vi "Universal_Stepping.vi"(7 "Initial Voltage (V)":dbl caption="Initial Value", 9 "Voltage Step (V)":dbl=0.01 caption="Step Value", 10 "Final Voltage (V)":dbl=0.1 caption="Final Value", 11 "VISA resource name":refnum<visa-resource-name>) -> (1 "Ready":bool, 2 "Actual Voltage (V)":dbl caption="Actual Value" step=0.1)   [LabVIEW 2015]
panel:
  in  "Command":string="smua.source.leveli="
  out "Visa Command":string
  out "Increase/Decrease":string
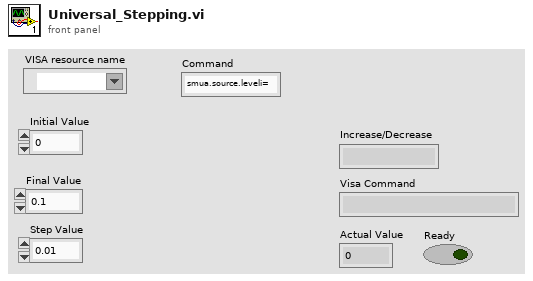
[diagram p1: front panel]
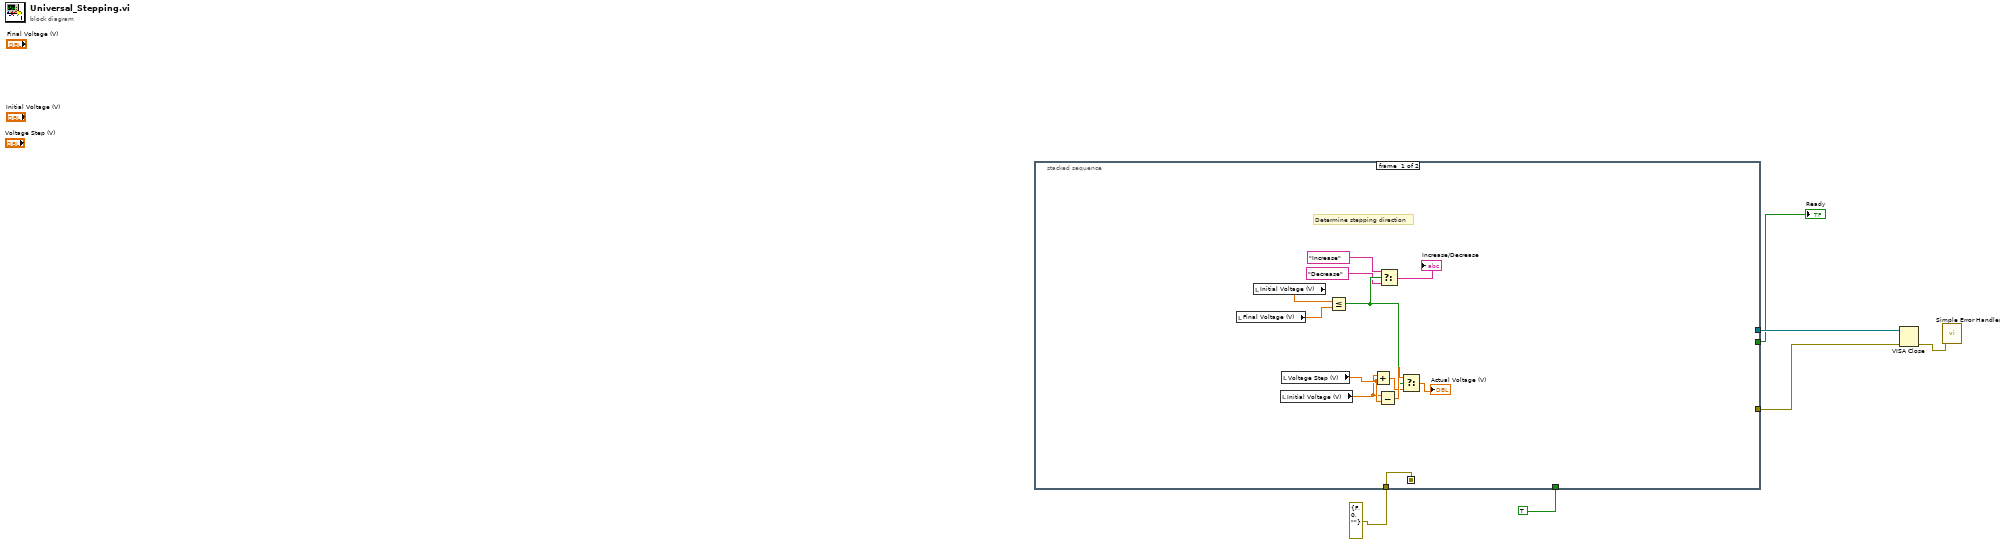
[diagram p0: block diagram]
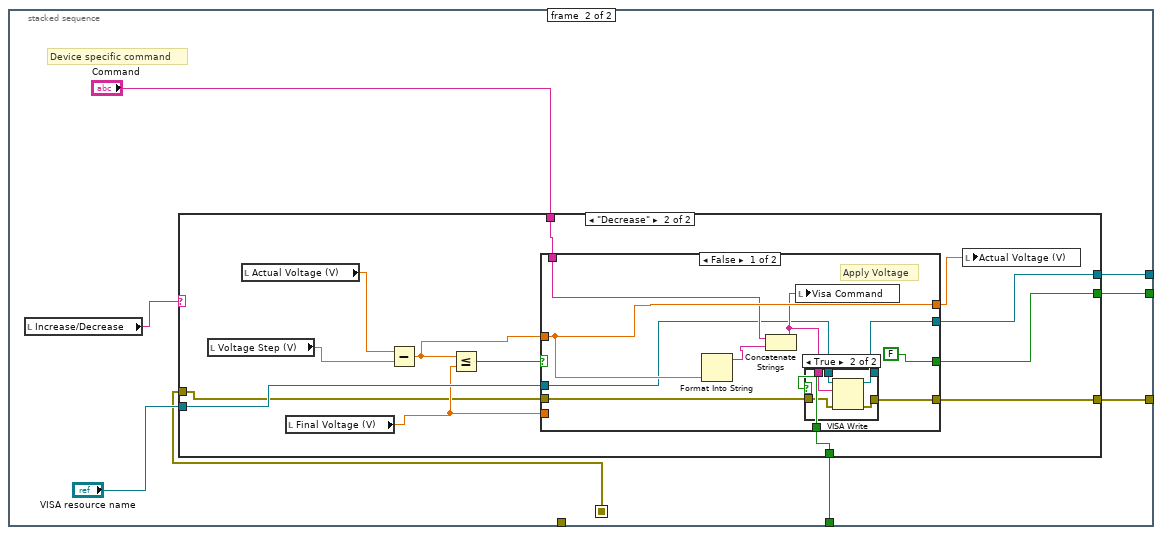
[diagram p2: hidden frame]
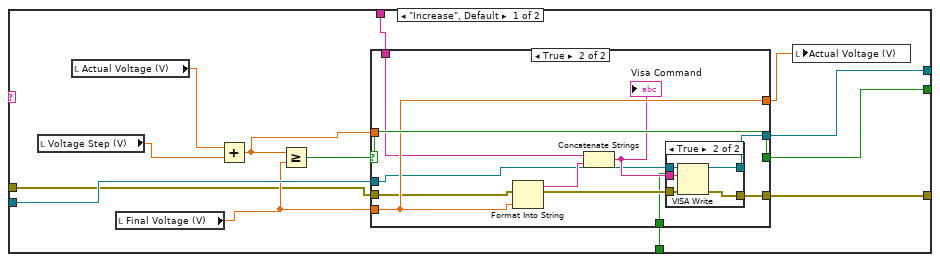
[diagram p3: hidden frame]
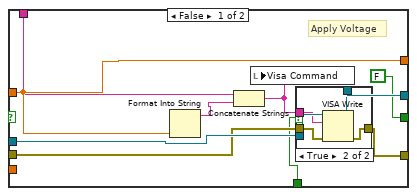
[diagram p4: hidden frame]
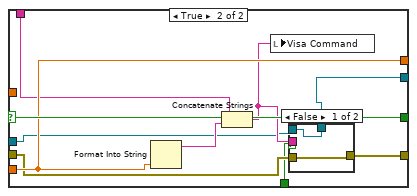
[diagram p8: hidden frame]
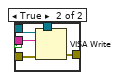
[diagram p9: hidden frame]
diagram:
  n1 = stacked-sequence {
    seq-local: [w18 _] -> [_ w24]
    tunnel: errorcluster {"status"=FALSE, "code"=0, "source"=""} ("error in (no error)") -> [w18 _]
    tunnel: [_ w25] -> w6
    tunnel: [_ w23] -> w3
    tunnel: [_ w22] -> w2
    tunnel: TRUE -> [_ w19]
    frame #0 {
      # "Determine stepping direction"
      n2 = local read "Final Voltage (V)"() -> (w8:dbl)
      n3 = local read "Initial Voltage (V)"() -> (w7:dbl)
      n4 = local read "Initial Voltage (V)"() -> (w12:dbl)
      n5 = local read "Voltage Step (V)"() -> (w13:dbl)
      n6 = Less Or Equal?(x=w7, y=w8) -> (x <= y?=w14:bool)
      n7 = Add(x=w12, y=w13) -> (x+y=w16:dbl)
      n8 = Subtract(x=w12, y=w13) -> (x-y=w17:dbl)
      n9 = Select(t="Increase", s=w14, f="Decrease") -> (s? t:f=→"Increase/Decrease":string)
      n10 = Select(t=w17, s=w14, f=w16) -> (s? t:f=→"Actual Voltage (V)":dbl)
    }
    frame #1 {
      # "Device specific command"
      n11 = local read "Increase/Decrease"() -> (w21:string)
      n12 = case shown="\"Decrease\"" w21 {
        tunnel: [w36 w83] -> w22
        tunnel: "VISA resource name" -> [w37 w84]
        tunnel: [w28 w78] -> w25
        tunnel: "Command" -> [w31 w77]
        tunnel: w24 -> [w30 w75]
        tunnel: [w29 w76] -> w23
        tunnel: w19 -> [w27 w74]
        frame "Increase", Default {
          n13 = local read "Voltage Step (V)"() -> (w35:dbl)
          n14 = local read "Actual Voltage (V)"() -> (w34:dbl)
          n15 = local read "Final Voltage (V)"() -> (w32:dbl)
          n16 = Add(x=w34, y=w35) -> (x+y=w39:dbl)
          n17 = Greater Or Equal?(x=w39, y=w32) -> (x >= y?=w38:bool)
          n18 = case shown="True" w38 {
            selector: w38 -> [_ w66]
            tunnel: [FALSE w66] -> w36
            tunnel: w39 -> [w48 _]
            tunnel: w37 -> [w46 w59]
            tunnel: [w48 w64] -> w33
            tunnel: w32 -> [_ w64]
            tunnel: w31 -> [w47 w63]
            tunnel: w30 -> [w44 w61]
            tunnel: [w43 w60] -> w29
            tunnel: [w45 w58] -> w28
            tunnel: w27 -> [w41 w57]
            frame False {
              # "Apply Voltage"
              n19 = Format Into String(w48) -> (resulting string=w49:string)  [unwired: 3 in, 1 out]
              n20 = Concatenate Strings(w47, w49) -> (w42:string)
              n21 = local write "Visa Command"(w42) -> ()
              n22 = case shown="True" w41 {
                tunnel: w46 -> [w50 w56]
                tunnel: [w50 w55] -> w45
                tunnel: w44 -> [w51 w54]
                tunnel: [w51 w53] -> w43
                tunnel: w42 -> [_ w52]
                frame False {
                }
                frame True {
                  n23 = VISA Write(VISA resource name=w56, write buffer=w52, error in (no error)=w54) -> (VISA resource name out=w55:refnum<visa-resource-name>, error out=w53:errorcluster)  [unwired: 1 out]
                }
              }
            }
            frame True {
              n24 = Format Into String(w64) -> (resulting string=w65:string)  [unwired: 3 in, 1 out]
              n25 = Concatenate Strings(w63, w65) -> (w62:string)
              "Visa Command" <- w62
              n26 = case shown="True" w57 {
                tunnel: w62 -> [_ w73]
                tunnel: w61 -> [w68 w72]
                tunnel: [w68 w71] -> w60
                tunnel: w59 -> [w67 w70]
                tunnel: [w67 w69] -> w58
                frame False {
                }
                frame True {
                  n27 = VISA Write(VISA resource name=w70, write buffer=w73, error in (no error)=w72) -> (VISA resource name out=w69:refnum<visa-resource-name>, error out=w71:errorcluster)  [unwired: 1 out]
                }
              }
            }
          }
          n28 = local write "Actual Voltage (V)"(w33) -> ()
        }
        frame "Decrease" {
          n29 = local read "Voltage Step (V)"() -> (w82:dbl)
          n30 = local read "Actual Voltage (V)"() -> (w81:dbl)
          n31 = local read "Final Voltage (V)"() -> (w79:dbl)
          n32 = Subtract(x=w81, y=w82) -> (x-y=w86:dbl)
          n33 = Less Or Equal?(x=w86, y=w79) -> (x <= y?=w85:bool)
          n34 = case shown="False" w85 {
            selector: w85 -> [_ w113]
            tunnel: [FALSE w113] -> w83
            tunnel: w86 -> [w94 _]
            tunnel: w84 -> [w91 w108]
            tunnel: [w90 w107] -> w78
            tunnel: [w94 w111] -> w80
            tunnel: w79 -> [_ w111]
            tunnel: w77 -> [w93 w110]
            tunnel: [w89 w105] -> w76
            tunnel: w75 -> [w88 w106]
            tunnel: w74 -> [w87 w104]
            frame False {
              # "Apply Voltage"
              n35 = Format Into String(w94) -> (resulting string=w95:string)  [unwired: 3 in, 1 out]
              n36 = Concatenate Strings(w93, w95) -> (w92:string)
              n37 = local write "Visa Command"(w92) -> ()
              n38 = case shown="True" w87 {
                tunnel: w92 -> [_ w103]
                tunnel: w91 -> [w97 w102]
                tunnel: [w97 w101] -> w90
                tunnel: [w98 w100] -> w89
                tunnel: w88 -> [w98 w99]
                frame False {
                }
                frame True {
                  n39 = VISA Write(VISA resource name=w102, write buffer=w103, error in (no error)=w99) -> (VISA resource name out=w101:refnum<visa-resource-name>, error out=w100:errorcluster)  [unwired: 1 out]
                }
              }
            }
            frame True {
              n40 = Format Into String(w111) -> (resulting string=w112:string)  [unwired: 3 in, 1 out]
              n41 = Concatenate Strings(w110, w112) -> (w109:string)
              n42 = local write "Visa Command"(w109) -> ()
              n43 = case shown="False" w104 {
                tunnel: w109 -> [_ w120]
                tunnel: w108 -> [w114 w119]
                tunnel: [w114 w118] -> w107
                tunnel: w106 -> [w115 w117]
                tunnel: [w115 w116] -> w105
                frame False {
                }
                frame True {
                  n44 = VISA Write(VISA resource name=w119, write buffer=w120, error in (no error)=w117) -> (VISA resource name out=w118:refnum<visa-resource-name>, error out=w116:errorcluster)  [unwired: 1 out]
                }
              }
            }
          }
          n45 = local write "Actual Voltage (V)"(w80) -> ()
        }
      }
    }
  }
  "Ready" <- w2
  n46 = VISA Close(VISA resource name=w6, error in (no error)=w3) -> (error out=w5:errorcluster)
  n47 = call <vilib>:"Simple Error Handler.vi"("error in (no error)"=w5) -> ()  [unwired: 4 in, 5 out]
